vi "Main.vi"() -> ()   [LabVIEW 2018]
doc: "This Continuous Measurement sample project is based on the Queued Message Handler template.\n\nThe Event Handling Loop generates messages based on user interface actions.\n\nThe Message Handling Loop processes messages generated by the Event Handling Loop, or by other messages. There are also Acquisition and Logging message handling loop subVIs, and a chart updating loop."
uses:
  Settings/Settings.ctl
  Acquisition/Hardware Configuration.ctl
  Acquisition/Signal Type.ctl
  Logging/Logging Configuration.ctl
  controls/UI Data.ctl
  controls/UI State.ctl
  support/Message Queue/Enqueue Message (Single).vi
  support/Message Queue/Enqueue Message (Array).vi
  <vilib>/Utility/error.llb/Error Cluster From Error Code.vi
  <vilib>/ErrorRing/Error Ring.xnode
  Acquisition/Acquisition.lvlib
  Logging/Logging.lvlib
  Settings/Settings.lvlib
  support/User Event - Stop/User Event - Stop.lvlib
  support/Message Queue/Message Queue.lvlib
  Settings/Settings Dialog.vi
panel:
  out "Data":waveform(dbl)[](graph)
  in  "Settings":bool
  in  "Start":bool
  in  "Stop":bool
  out "Status":string
  in  "Exit":bool
  # "Continuous Measurement Data Logger"
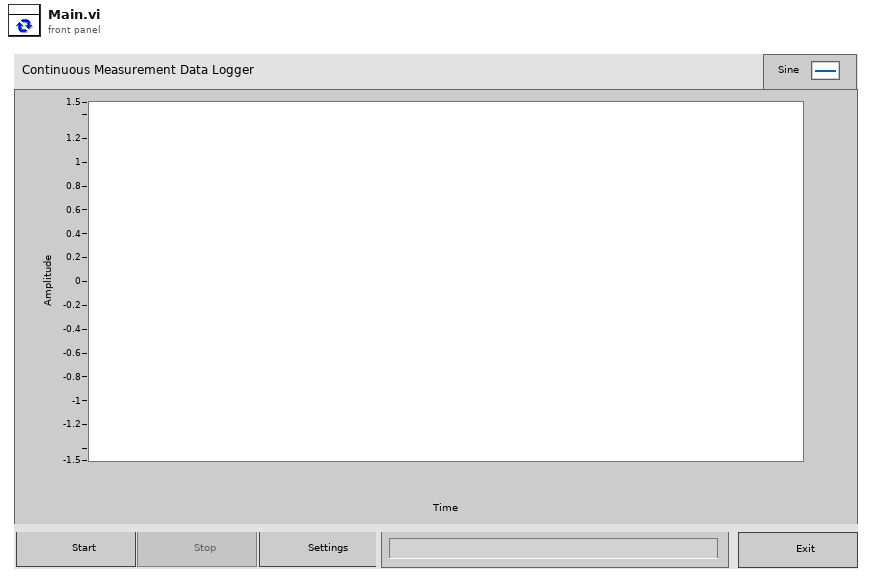
[diagram p1: front panel]
types:
  T1 = typedef "UI State.ctl" = enum16{"Idle", "Acquiring and Logging", "Waiting for Exit", "Waiting for Exit (Acq Stopped)", "Waiting for Exit (Log Stopped)", "Waiting for Stop", "Waiting for Stop (Acq Stopped)", "Waiting for Stop (Log Stopped)"}
  T2 = typedef "UI Data.ctl" = cluster{"Start Ref":refnum<vi>, "Stop Ref":refnum<vi>, "Settings Ref":refnum<vi>, "Exit Ref":refnum<vi>, "Status Ref":refnum<vi>, "Data Ref":refnum<vi>}
  T3 = typedef "Settings.lvlib/Settings.ctl" = cluster{"Hardware Configuration":T4, "Logging Configuration":T6}
  T4 = typedef "Acquisition.lvlib/Hardware Configuration.ctl" = cluster{"HW Refnum <Replace Me>":string, "Signal Type <Replace Me>":T5}
  T5 = typedef "Acquisition.lvlib/Signal Type.ctl" = enum16{"Sine Wave", "Square with Noise"}
  T6 = typedef "Logging.lvlib/Logging Configuration.ctl" = cluster{"Log File Base Path":path, "TDMS File Reference":refnum<k34>}
  T7 = typedef "Message Queue.lvlib/All Message Queues.ctl" = cluster{"UI":refnum<queue>, "Acquisition":refnum<queue>, "Logging":refnum<queue>}
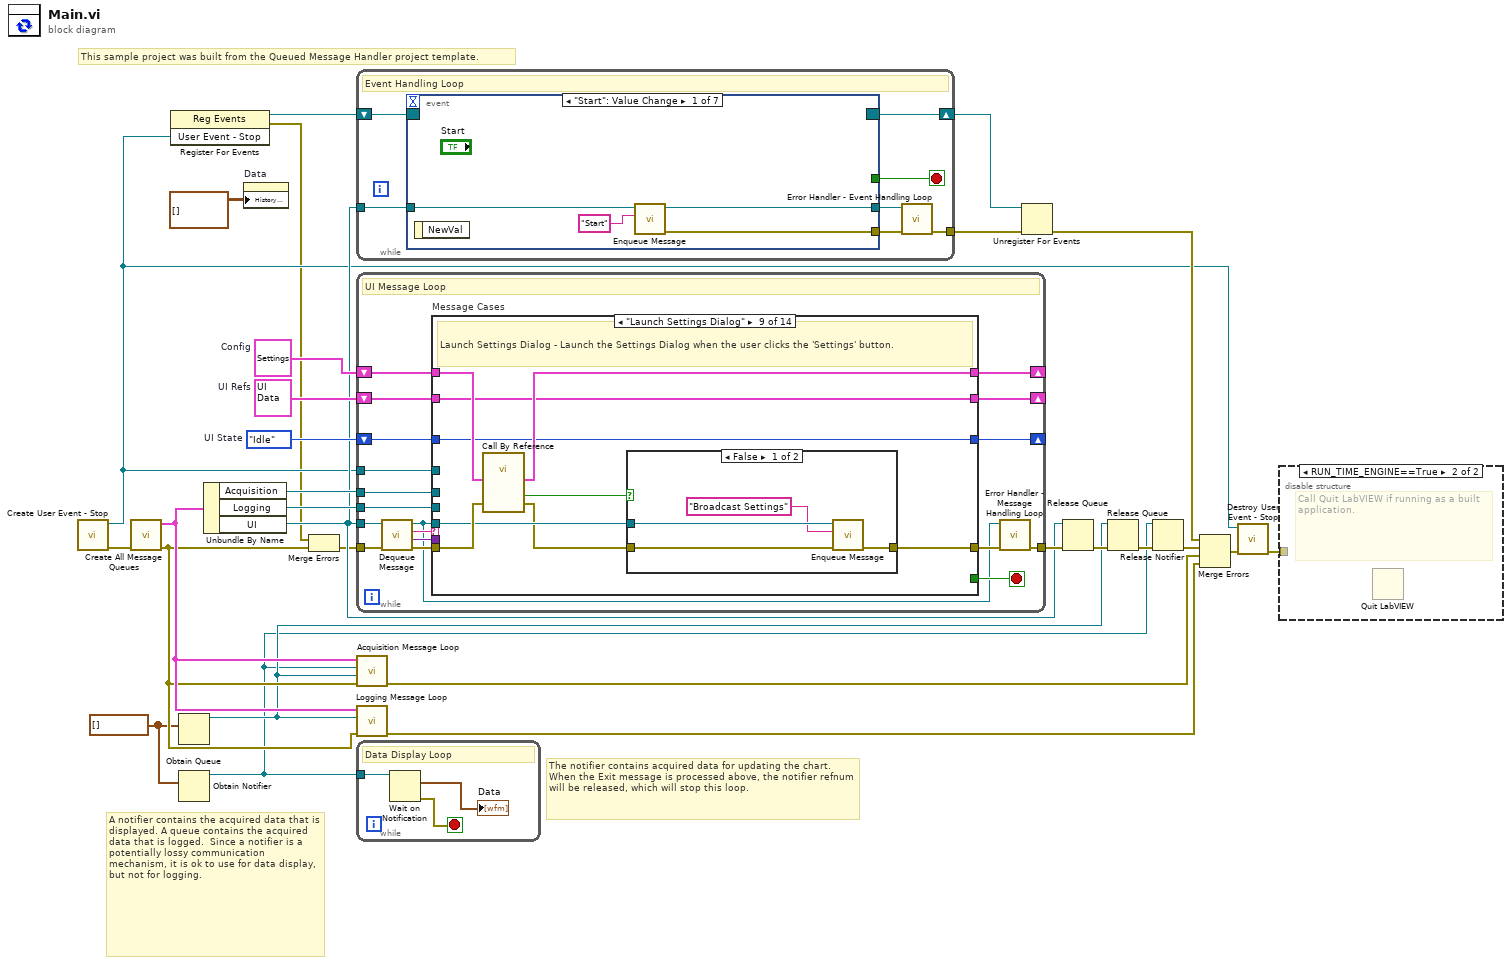
[diagram p0: block diagram]
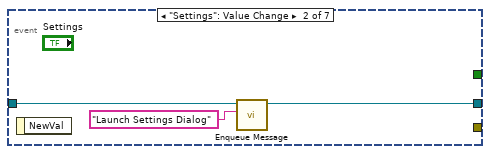
[diagram p3: hidden frame]
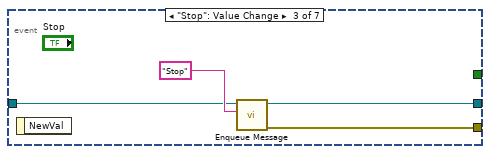
[diagram p4: hidden frame]
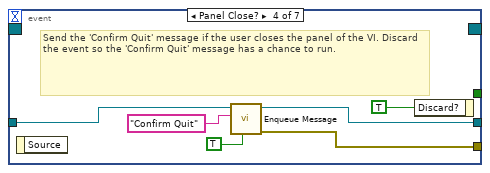
[diagram p5: hidden frame]
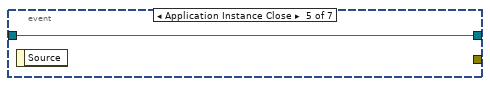
[diagram p6: hidden frame]
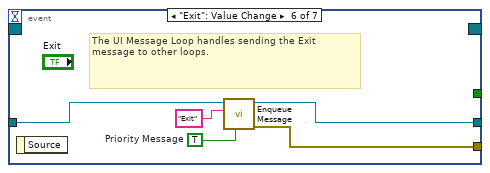
[diagram p7: hidden frame]
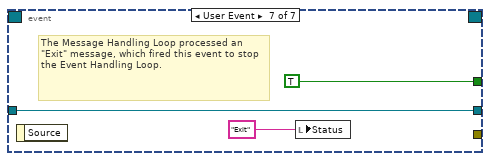
[diagram p8: hidden frame]
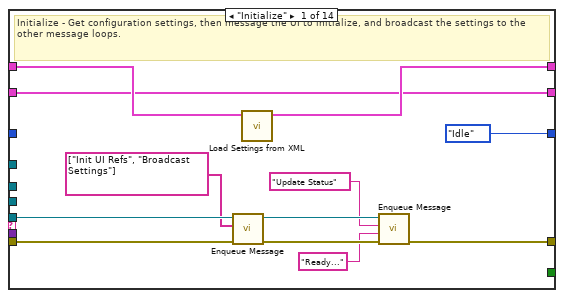
[diagram p9: hidden frame]
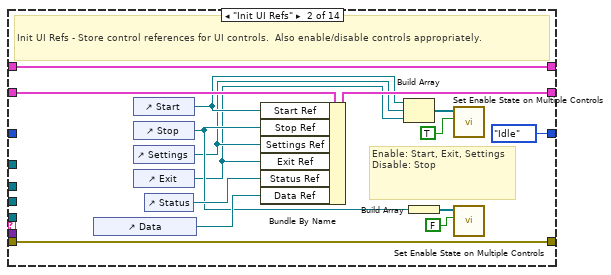
[diagram p10: hidden frame]
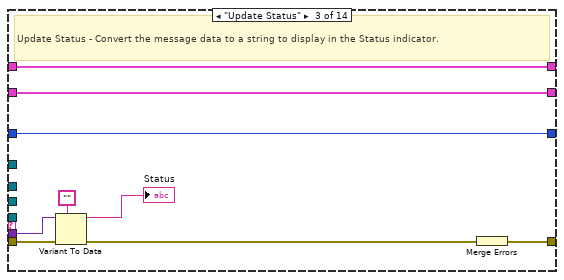
[diagram p11: hidden frame]
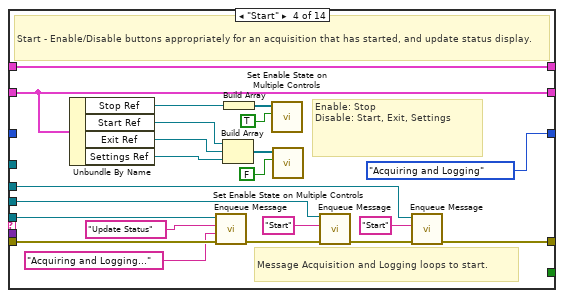
[diagram p12: hidden frame]
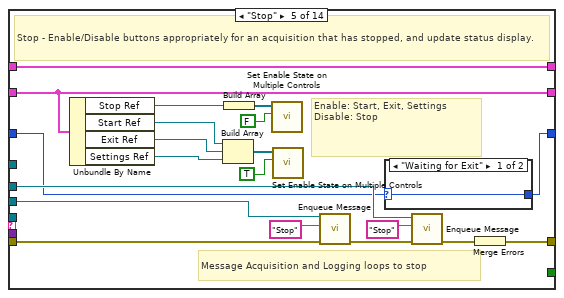
[diagram p13: hidden frame]
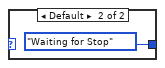
[diagram p14: hidden frame]
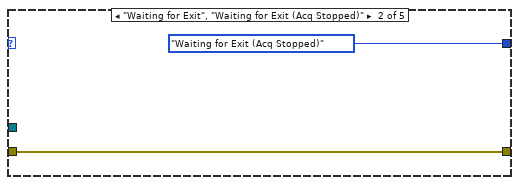
[diagram p16: hidden frame]
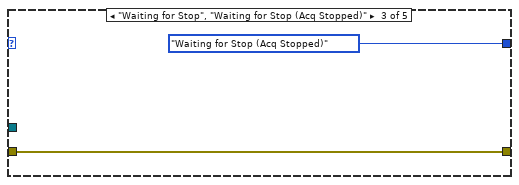
[diagram p17: hidden frame]
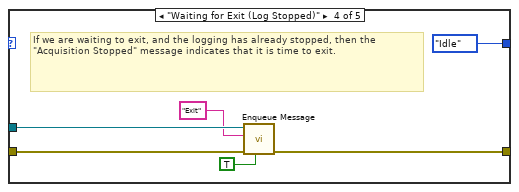
[diagram p18: hidden frame]
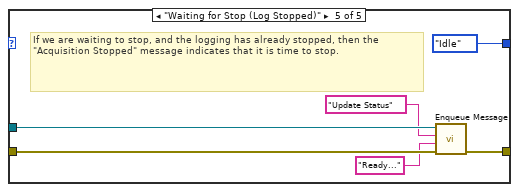
[diagram p19: hidden frame]
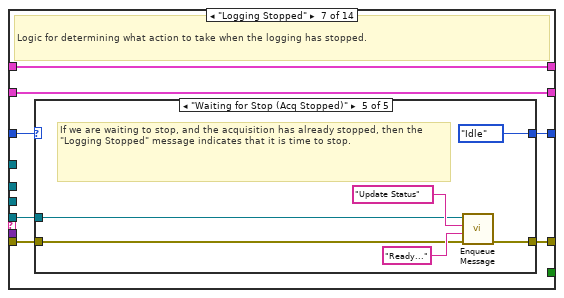
[diagram p20: hidden frame]
diagram:
  w15 = UI_State."Idle"  # UI State
  w6 = waveform(dbl)[] []
  w18 = T2 {"Start Ref"=refnum, "Stop Ref"=refnum, "Settings Ref"=refnum, "Exit Ref"=refnum, "Status Ref"=refnum, "Data Ref"=refnum}  # UI Refs
  w21 = T3 {"Hardware Configuration"={"HW Refnum <Replace Me>"="", "Signal Type <Replace Me>"=enum."Sine Wave"}, "Logging Configuration"={"Log File Base Path"=path "", "TDMS File Reference"=refnum}}  # Config
  # "This sample project was built from the Queued Message Handler project template."
  # "A notifier contains the acquired data that is displayed. A queue contains the acquired data that is logged.  Since a notifier is a potentially lossy communication mechanism, it is ok to use for data display, but not for logging."
  # "The notifier contains acquired data for updating the chart. When the Exit message is processed above, the notifier refnum will be released, which will stop this loop."
  n1 = call "Create User Event - Stop.vi"() -> ("error out"=w25:errorcluster, "User Event - Stop"=w4:refnum<user-event>)  [unwired: 10 in]
  n2 = call "Create All Message Queues.vi"("error in (no error)"=w25) -> ("error out"=w22:errorcluster, "Message Queues out"=w24:T7)  [unwired: 9 in]
  n3 = register-events(w4) -> (reference out=w5:refnum<event-registration>, error out=w2:errorcluster)  [unwired: 2 in]
  n4 = Obtain Queue(element data type=w6) -> (queue out=w8:refnum<queue>)  [unwired: 4 in, 2 out]
  n5 = Obtain Notifier(notification data type=w6) -> (notifier out=w7:refnum<notifier>)  [unwired: 3 in, 2 out]
  n6 = Unbundle By Name(w24) -> ("Acquisition"=w17:refnum<queue>, "Logging"=w16:refnum<queue>, "UI"=w13:refnum<queue>)
  n7 = property on="Data" class="WFChart (strict)"("History Data"=waveform(dbl)[][] []) -> ()  [unwired: 2 in, 2 out]
  n8 = Merge Errors(w2, w22) -> (w3:errorcluster)
  n9 = while {
    tunnel: w13 -> [w34]
    tunnel: [w31] -> w27
    shift-right: [w33] -> w19
    shift-left: w5 -> [w35]
    stop <- w32 stop-if-true
    # "Event Handling Loop"
    n10 = event shown="[0] \"Start\": Value Change" {
      selector: w35 -> [_ _ _ _ _ _ _]
      dyn-events: [_ _ _ _ _ _ _] -> w33
      timeout: _ -> [_ _ _ _ _ _ _]
      tunnel: [_ _ _ _ _ _ TRUE ("Discard?")] -> w32
      tunnel: w34 -> [w39 w41 w45 w50 w53 w55 w59]
      tunnel: [w37 _ w44 w48 _ w58 _] -> w30
      tunnel: [w36 w40 w43 w49 w53 w54 w59] -> w29
      event "Start": Value Change {
        n11 = event-data() -> ()  [unwired: 1 in, 1 out]
        n12 = call-poly "Enqueue Message.vi"("Message"="Start", "Message Queue"=w39) -> ("error out"=w37:errorcluster, "dup Message Queue"=w36:refnum<queue>)  [unwired: 8 in]
      }
      event "Settings": Value Change {
        n13 = event-data() -> ()  [unwired: 1 in, 1 out]
        n14 = call-poly "Enqueue Message.vi"("Message"="Launch Settings Dialog", "Message Queue"=w41) -> ("dup Message Queue"=w40:refnum<queue>)  [unwired: 8 in, 1 out]
      }
      event "Stop": Value Change {
        n15 = event-data() -> ()  [unwired: 1 in, 1 out]
        n16 = call-poly "Enqueue Message.vi"("Message"="Stop", "Message Queue"=w45) -> ("error out"=w44:errorcluster, "dup Message Queue"=w43:refnum<queue>)  [unwired: 8 in]
      }
      event Panel Close? {
        # "Send the 'Confirm Quit' message if the user closes the panel of the VI. Discard the event so the 'Confirm Quit' message has a chance to run."
        n17 = event-data() -> ()  [unwired: 1 in, 1 out]
        n18 = call-poly "Enqueue Message.vi"("Priority Message? (F)"=TRUE, "Message"="Confirm Quit", "Message Queue"=w50) -> ("error out"=w48:errorcluster, "dup Message Queue"=w49:refnum<queue>)  [unwired: 7 in]
        n19 = event-data("Discard?"=TRUE) -> ()  [unwired: 1 in, 1 out]
      }
      event Application Instance Close {
        n20 = event-data() -> ()  [unwired: 1 in, 1 out]
      }
      event "Exit": Value Change {
        w56 = TRUE  # Priority Message
        # "The UI Message Loop handles sending the Exit message to other loops."
        n21 = event-data() -> ()  [unwired: 1 in, 1 out]
        n22 = call-poly "Enqueue Message.vi"("Priority Message? (F)"=w56, "Message"="Exit", "Message Queue"=w55) -> ("error out"=w58:errorcluster, "dup Message Queue"=w54:refnum<queue>)  [unwired: 7 in]
      }
      event User Event {
        # "The Message Handling Loop processed an \"Exit\" message, which fired this event to stop the Event Handling Loop."
        n23 = event-data() -> ()  [unwired: 1 in, 1 out]
        n24 = local write "Status"("Exit" ("Exit String")) -> ()
      }
    }
    n25 = call "Error Handler - Event Handling Loop.vi"("error in (no error)"=w30, "Message Queue"=w29) -> ("dup error in"=w31:errorcluster)  [unwired: 8 in, 1 out]
  }
  n26 = while {
    tunnel: w13 -> [w73]
    tunnel: w4 -> [w78]
    shift-right: [w72] -> _
    shift-left: w21 -> [w71]
    shift-right: [w69] -> _
    shift-left: w18 -> [w70]
    tunnel: w17 -> [w68]
    tunnel: w16 -> [w67]
    shift-right: [w62] -> _
    shift-left: w15 -> [w63]
    tunnel: w3 -> [w77]
    tunnel: [w66] -> w28
    stop <- w79 stop-if-true
    # "UI Message Loop"
    n27 = call "Dequeue Message.vi"("error in (no error)"=w77, "Message Queue"=w73) -> ("error out"=w76:errorcluster, "Message Data"=w74:variant, "Message"=w75:string, "dup Message Queue"=w64:refnum<queue>)  [unwired: 6 in]
    n28 = case "Message Cases" shown="\"Launch Settings Dialog\"" w75 {
      selector: w75 -> [_ _ _ _ _ _ _ _ _ _ _ _ _ w295]
      tunnel: w64 -> [w83 _ _ w137 _ w162 w187 _ w227 _ w248 _ _ _]
      tunnel: w76 -> [w82 w106 w114 w136 w156 w163 w188 w215 w229 w236 w247 w276 w293 _]
      tunnel: [w87 w106 w115 w119 w157 w160 w185 w221 w222 w239 w246 w286 w292 w294] -> w65
      tunnel: [_ _ _ _ _ _ _ _ _ _ _ TRUE _ _] -> w79
      tunnel: w74 -> [_ _ w113 _ _ _ _ _ _ w240 _ w274 _ _]
      tunnel: w78 -> [_ _ _ _ _ _ _ _ _ _ _ w287 _ _]
      tunnel: [w90 w105 w109 w135 w155 w166 w191 w219 w226 w244 w251 w285 w291 w298] -> w72
      tunnel: w71 -> [w91 w105 w109 w135 w155 w166 w191 w219 w230 w244 w251 w285 w291 w298]
      tunnel: w70 -> [w84 w104 w108 w132 w154 w165 w190 w213 w224 w243 w250 w284 w290 w297]
      tunnel: [w84 w101 w108 w132 w154 w165 w190 w213 w224 w243 w250 w284 w290 w297] -> w69
      tunnel: w68 -> [_ _ _ w118 w141 _ _ w212 _ _ _ w283 _ _]
      tunnel: w67 -> [_ _ _ w121 w144 _ _ w211 _ _ _ w282 _ _]
      tunnel: w63 -> [_ _ w107 _ w138 w164 w189 w210 w223 w238 w249 _ w289 w296]
      tunnel: [UI_State."Idle" ("UI State") UI_State."Idle" ("UI State") w107 UI_State."Acquiring and Logging" ("UI State") w139 w161 w186 w210 w223 w238 w245 UI_State."Idle" ("UI State") w289 w296] -> w62
      frame "Initialize" {
        # "Initialize - Get configuration settings, then message the UI to initialize, and broadcast the settings to the other message loops."
        n29 = call-poly "Enqueue Message.vi"("error in (no error)"=w82, "Message Array"=string[] ["Init UI Refs", "Broadcast Settings"], "Message Queue"=w83) -> ("error out"=w89:errorcluster, "dup Message Queue"=w88:refnum<queue>)  [unwired: 7 in]
        n30 = call "Load Settings from XML.vi"("Settings in"=w91) -> ("Settings out"=w90:T3)  [unwired: 9 in, 1 out]
        n31 = call-poly "Enqueue Message.vi"("error in (no error)"=w89, "Message Data"="Ready..." ("Ready..."), "Message"="Update Status", "Message Queue"=w88) -> ("error out"=w87:errorcluster)  [unwired: 6 in, 1 out]
      }
      frame "Init UI Refs" {
        # "Enable: Start, Exit, Settings\nDisable: Stop"
        # "Init UI Refs - Store control references for UI controls.  Also enable/disable controls appropriately."
        n32 = control-ref of="Data"() -> (w102:refnum<vi>)
        n33 = control-ref of="Start"() -> (w95:refnum<vi>)
        n34 = control-ref of="Stop"() -> (w96:refnum<vi>)
        n35 = control-ref of="Settings"() -> (w94:refnum<vi>)
        n36 = control-ref of="Exit"() -> (w93:refnum<vi>)
        n37 = control-ref of="Status"() -> (w103:refnum<vi>)
        n38 = Bundle By Name(cluster=w104, "Start Ref"=w95, "Stop Ref"=w96, "Settings Ref"=w94, "Exit Ref"=w93, "Status Ref"=w103, "Data Ref"=w102) -> (w101:T2)
        n39 = Build Array(w95, w94, w93) -> (w99:refnum<vi>[])
        n40 = Build Array(w96) -> (w98:refnum<vi>[])
        n41 = call "Set Enable State on Multiple Controls.vi"("Enable?"=TRUE, "Controls"=w99) -> ()  [unwired: 10 in]
        n42 = call "Set Enable State on Multiple Controls.vi"("Enable?"=FALSE, "Controls"=w98) -> ()  [unwired: 10 in]
      }
      frame "Update Status" {
        # "Update Status - Convert the message data to a string to display in the Status indicator."
        n43 = Variant To Data(error in=w114, type="", Variant=w113) -> (data=→"Status":string, error out=w111:errorcluster)
        n44 = Merge Errors(w111) -> (w115:errorcluster)
      }
      frame "Start" {
        # "Message Acquisition and Logging loops to start."
        # "Enable: Stop\nDisable: Start, Exit, Settings"
        # "Start - Enable/Disable buttons appropriately for an acquisition that has started, and update status display."
        n45 = Unbundle By Name(w132) -> ("Stop Ref"=w127:refnum<vi>, "Start Ref"=w126:refnum<vi>, "Exit Ref"=w125:refnum<vi>, "Settings Ref"=w124:refnum<vi>)
        n46 = call-poly "Enqueue Message.vi"("error in (no error)"=w136, "Message Data"="Acquiring and Logging..." ("Acquiring and Logging..."), "Message"="Update Status", "Message Queue"=w137) -> ("error out"=w123:errorcluster)  [unwired: 6 in, 1 out]
        n47 = Build Array(w126, w125, w124) -> (w130:refnum<vi>[])
        n48 = Build Array(w127) -> (w129:refnum<vi>[])
        n49 = call "Set Enable State on Multiple Controls.vi"("Enable?"=TRUE, "Controls"=w129) -> ()  [unwired: 10 in]
        n50 = call "Set Enable State on Multiple Controls.vi"("Enable?"=FALSE, "Controls"=w130) -> ()  [unwired: 10 in]
        n51 = call-poly "Enqueue Message.vi"("error in (no error)"=w123, "Message"="Start", "Message Queue"=w121) -> ("error out"=w120:errorcluster)  [unwired: 7 in, 1 out]
        n52 = call-poly "Enqueue Message.vi"("error in (no error)"=w120, "Message"="Start", "Message Queue"=w118) -> ("error out"=w119:errorcluster)  [unwired: 7 in, 1 out]
      }
      frame "Stop" {
        # "Message Acquisition and Logging loops to stop"
        # "Enable: Start, Exit, Settings\nDisable: Stop"
        # "Stop - Enable/Disable buttons appropriately for an acquisition that has stopped, and update status display."
        n53 = Unbundle By Name(w154) -> ("Stop Ref"=w149:refnum<vi>, "Start Ref"=w148:refnum<vi>, "Exit Ref"=w147:refnum<vi>, "Settings Ref"=w146:refnum<vi>)
        n54 = Build Array(w148, w147, w146) -> (w152:refnum<vi>[])
        n55 = Build Array(w149) -> (w151:refnum<vi>[])
        n56 = call "Set Enable State on Multiple Controls.vi"("Enable?"=FALSE, "Controls"=w151) -> ()  [unwired: 10 in]
        n57 = call "Set Enable State on Multiple Controls.vi"("Enable?"=TRUE, "Controls"=w152) -> ()  [unwired: 10 in]
        n58 = call-poly "Enqueue Message.vi"("error in (no error)"=w156, "Message"="Stop", "Message Queue"=w144) -> ("error out"=w143:errorcluster)  [unwired: 7 in, 1 out]
        n59 = case shown="\"Waiting for Exit\"" w138 {
          selector: w138 -> [w158 _]
          tunnel: [w158 UI_State."Waiting for Stop" ("UI State")] -> w139
          frame "Waiting for Exit" {
          }
          frame Default {
          }
        }
        n60 = call-poly "Enqueue Message.vi"("error in (no error)"=w143, "Message"="Stop", "Message Queue"=w141) -> ("error out"=w142:errorcluster)  [unwired: 7 in, 1 out]
        n61 = Merge Errors(w142) -> (w157:errorcluster)
      }
      frame "Acquisition Stopped" {
        # "Logic for determining what action to take when the acquisition has stopped."
        n62 = case shown="Default" w164 {
          selector: w164 -> [w168 _ _ _ _]
          tunnel: w163 -> [w167 w170 w172 w178 w184]
          tunnel: w162 -> [_ _ _ w176 w181]
          tunnel: [w168 UI_State."Waiting for Exit (Acq Stopped)" ("UI State") UI_State."Waiting for Stop (Acq Stopped)" ("UI State") UI_State."Idle" ("UI State") UI_State."Idle" ("UI State")] -> w161
          tunnel: [w167 w170 w172 w177 w182] -> w160
          frame Default {
          }
          frame "Waiting for Exit", "Waiting for Exit (Acq Stopped)" {
          }
          frame "Waiting for Stop", "Waiting for Stop (Acq Stopped)" {
          }
          frame "Waiting for Exit (Log Stopped)" {
            # "If we are waiting to exit, and the logging has already stopped, then the \"Acquisition Stopped\" message indicates that it is time to exit."
            n63 = call-poly "Enqueue Message.vi"("Priority Message? (F)"=TRUE, "error in (no error)"=w178, "Message"="Exit", "Message Queue"=w176) -> ("error out"=w177:errorcluster)  [unwired: 6 in, 1 out]
          }
          frame "Waiting for Stop (Log Stopped)" {
            # "If we are waiting to stop, and the logging has already stopped, then the \"Acquisition Stopped\" message indicates that it is time to stop."
            n64 = call-poly "Enqueue Message.vi"("error in (no error)"=w184, "Message Data"="Ready..." ("Ready..."), "Message"="Update Status", "Message Queue"=w181) -> ("error out"=w182:errorcluster)  [unwired: 6 in, 1 out]
          }
        }
      }
      frame "Logging Stopped" {
        # "Logic for determining what action to take when the logging has stopped."
        n65 = case shown="\"Waiting for Stop (Acq Stopped)\"" w189 {
          selector: w189 -> [w193 _ _ _ _]
          tunnel: w188 -> [w192 w195 w197 w203 w206]
          tunnel: w187 -> [_ _ _ w201 w205]
          tunnel: [w193 UI_State."Waiting for Exit (Log Stopped)" ("UI State") UI_State."Waiting for Stop (Log Stopped)" ("UI State") UI_State."Idle" ("UI State") UI_State."Idle" ("UI State")] -> w186
          tunnel: [w192 w195 w197 w202 w204] -> w185
          frame Default {
          }
          frame "Waiting for Exit", "Waiting for Exit (Log Stopped)" {
          }
          frame "Waiting for Stop", "Waiting for Stop (Log Stopped)" {
          }
          frame "Waiting for Exit (Acq Stopped)" {
            # "If we are waiting to exit, and the acquisition has already stopped, then the \"Logging Stopped\" message indicates that it is time to exit."
            n66 = call-poly "Enqueue Message.vi"("Priority Message? (F)"=TRUE, "error in (no error)"=w203, "Message"="Exit", "Message Queue"=w201) -> ("error out"=w202:errorcluster)  [unwired: 6 in, 1 out]
          }
          frame "Waiting for Stop (Acq Stopped)" {
            # "If we are waiting to stop, and the acquisition has already stopped, then the \"Logging Stopped\" message indicates that it is time to stop."
            n67 = call-poly "Enqueue Message.vi"("error in (no error)"=w206, "Message Data"="Ready..." ("Ready..."), "Message"="Update Status", "Message Queue"=w205) -> ("error out"=w204:errorcluster)  [unwired: 6 in, 1 out]
          }
        }
      }
      frame "Broadcast settings" {
        w214 = "Update Settings" ("Message")
        # "Broadcast settings - Send the 'Update Settings' message to the Logging and Acquisition message loops."
        n68 = Unbundle By Name(w219) -> ("Hardware Configuration"=w218:T4, "Logging Configuration"=w217:T6)
        n69 = call-poly "Enqueue Message.vi"("Message Data"=w218, "Message"=w214, "Message Queue"=w212) -> ("error out"=w220:errorcluster)  [unwired: 7 in, 1 out]
        n70 = call-poly "Enqueue Message.vi"("error in (no error)"=w220, "Message Data"=w217, "Message"=w214, "Message Queue"=w211) -> ("error out"=w216:errorcluster)  [unwired: 6 in, 1 out]
        n71 = Merge Errors(w216, w215) -> (w221:errorcluster)
      }
      frame "Launch Settings Dialog" {
        # "Launch Settings Dialog - Launch the Settings Dialog when the user clicks the 'Settings' button."
        n72 = call-by-ref "?"("error in (no error)"=w229, "Settings in"=w230) -> ("error out"=w225:errorcluster, "Cancelled?"=w228:bool, "Settings out"=w226:T3)  [unwired: 8 in, 3 out]
        n73 = case shown="False" w228 {
          tunnel: w227 -> [w234 _]
          tunnel: w225 -> [w233 w235]
          tunnel: [w232 w235] -> w222
          frame False {
            n74 = call-poly "Enqueue Message.vi"("error in (no error)"=w233, "Message"="Broadcast Settings", "Message Queue"=w234) -> ("error out"=w232:errorcluster)  [unwired: 7 in, 1 out]
          }
          frame True {
          }
        }
      }
      frame "Error" {
        # "Error - Display an error dialog. This message is sent by the \"Error Handler\" VIs at the end of other loops in this application."
        n75 = Variant To Data(error in=w236, type=errorcluster {"status"=FALSE, "code"=0, "source"=""} ("error constant"), Variant=w240) -> (data=w237:errorcluster, error out=w241:errorcluster)
        n76 = call <vilib>:"Simple Error Handler.vi"("error in (no error)"=w237) -> ()  [unwired: 4 in, 5 out]
        n77 = Merge Errors(w241) -> (w239:errorcluster)
      }
      frame "Confirm Quit" {
        # "Confirm Quit - Message that can confirm whether or not the user wants to exit the application."
        n78 = case shown="\"Acquiring and Logging\"" w249 {
          tunnel: w248 -> [w257 w261]
          tunnel: w247 -> [w256 w260]
          tunnel: [w255 w259] -> w246
          tunnel: [UI_State."Idle" ("UI State") w258] -> w245
          frame Default {
            # "If 'Confirm Quit' comes in while the system is idle, there is no need for a confirmation message."
            n79 = call-poly "Enqueue Message.vi"("Priority Message? (F)"=TRUE, "error in (no error)"=w256, "Message"="Exit", "Message Queue"=w257) -> ("error out"=w255:errorcluster)  [unwired: 6 in, 1 out]
          }
          frame "Acquiring and Logging" {
            n80 = Two Button Dialog(message="Are you sure you want to quit while the acquisition is running?" ("Confirm Quit Message"), 1:"No" ("No"), 2:"Yes" ("Yes")) -> (T button?=w262:bool)
            n81 = case shown="True" w262 {
              tunnel: w261 -> [_ w271]
              tunnel: w260 -> [w267 w272]
              tunnel: [w267 w270] -> w259
              tunnel: [UI_State."Acquiring and Logging" ("UI State") UI_State."Waiting for Exit" ("UI State")] -> w258
              frame False {
                # "User did not want to quit."
              }
              frame True {
                n82 = call-poly "Enqueue Message.vi"("error in (no error)"=w272, "Message"="Stop", "Message Queue"=w271) -> ("error out"=w270:errorcluster)  [unwired: 7 in, 1 out]
              }
            }
          }
        }
      }
      frame "Exit" {
        w278 = TRUE ("Priority Message? (F)")
        w279 = "Exit" ("Message")
        # "Popup an error dialog if 'Exit' was called as a result of an error."
        # "Stop the VI"
        # "Exit - Send Exit messages to the Acquisition and Logging loops, and fire the user event to stop the Event Handling Loop."
        n83 = Variant To Data(type=errorcluster {"status"=FALSE, "code"=0, "source"=""} ("error constant"), Variant=w274) -> (data=w273:errorcluster)  [unwired: 1 in, 1 out]
        n84 = call <vilib>:"Simple Error Handler.vi"("error in (no error)"=w273) -> ()  [unwired: 4 in, 5 out]
        n85 = call-poly "Enqueue Message.vi"("Priority Message? (F)"=w278, "error in (no error)"=w276, "Message"=w279, "Message Queue"=w283) -> ("error out"=w280:errorcluster)  [unwired: 6 in, 1 out]
        n86 = call-poly "Enqueue Message.vi"("Priority Message? (F)"=w278, "error in (no error)"=w280, "Message"=w279, "Message Queue"=w282) -> ("error out"=w277:errorcluster)  [unwired: 6 in, 1 out]
        n87 = call "Fire User Event - Stop.vi"("error in (no error)"=w277, "User Event - Stop"=w287) -> ("error out"=w286:errorcluster)  [unwired: 9 in]
      }
      frame "---Copy This Frame---" {
        # "Duplicate this frame when creating new messages.  Change this comment in the duplicated frame to describe this message."
        n88 = Merge Errors(w293) -> (w292:errorcluster)
      }
      frame Default {
        # "'Default' case only runs if there is a message that isn't defined in any of the other cases.  Output a programming error."
        n89 = xnode "Error Ring"("parameter 0"=w295) -> ("error out"=w294:errorcluster)
      }
    }
    n90 = call "Error Handler - Message Handling Loop.vi"("error in (no error)"=w65, "Message Queue"=w64) -> ("dup error in"=w66:errorcluster)  [unwired: 8 in, 1 out]
  }
  n91 = call "Acquisition Message Loop.vi"("error in (no error)"=w22, "Data Queue"=w8, "Data Notifier"=w7, "Message Queues"=w24) -> ("error out"=w26:errorcluster)  [unwired: 7 in]
  n92 = call "Logging Message Loop.vi"("error in (no error)"=w22, "Data Queue"=w8, "Message Queues"=w24) -> ("error out"=w23:errorcluster)  [unwired: 8 in]
  n93 = while "Data Display Loop" {
    tunnel: w7 -> [w308]
    stop <- w306 stop-if-true
    # "Data Display Loop"
    n94 = Wait on Notification(notifier=w308) -> (notification=→"Data":waveform(dbl)[], error out=w306:errorcluster)  [unwired: 3 in, 2 out]
  }
  n95 = Unregister For Events(event registration refnum=w19, error in=w27) -> (error out=w20:errorcluster)
  n96 = Release Queue(queue=w13, error in (no error)=w28) -> (error out=w11:errorcluster)  [unwired: 1 in, 2 out]
  n97 = Release Queue(queue=w8, error in (no error)=w11) -> (error out=w10:errorcluster)  [unwired: 1 in, 2 out]
  n98 = Release Notifier(notifier=w7, error in (no error)=w10) -> (error out=w9:errorcluster)  [unwired: 1 in, 2 out]
  n99 = Merge Errors(w20, w9, w26, w23) -> (w14:errorcluster)
  n100 = call "Destroy User Event - Stop.vi"("error in (no error)"=w14, "User Event - Stop"=w4) -> ("error out"=w12:errorcluster)  [unwired: 9 in]
  n101 = disable-structure shown="RUN_TIME_ENGINE==True" {
    disable-tunnel: w12 -> [_ _]
    frame condition #0 (active) {
    }
    frame condition #1 {
      # "Call Quit LabVIEW if running as a built application."
      n102 = Quit LabVIEW() -> ()  [unwired: 1 in]
    }
  }
